vi "Database Recordset Open.vi"(6 "LockType":i32(ring)=-1 items=["adLockUnspecified"=-1, "adLockReadOnly"=1, "adLockPessimistic"=2, "adLockOptimistic"=3, "adLockBatchOptimistic"=4], 7 "CursorType":i32(ring)=-1 items=["adOpenUnspecified"=-1, "adOpenForwardOnly"=0, "adOpenKeyset"=1, "adOpenDynamic"=2, "adOpenStatic"=3], 8 "error in (no error)":errorcluster caption="错误输入（无错误）", 9 "Options":i32, 10 "Command Text":string, 11 "Database Recordset 输入":refnum<class "Database Recordset.lvclass"> caption="DNL_LabVIEW Object in") -> (0 "error out":errorcluster caption="错误输出", 3 "Database Recordset 输出":refnum<class "Database Recordset.lvclass"> caption="DNL_LabVIEW Object out")   [LabVIEW 2011, in "Database Recordset.lvclass"]
uses:
  Database Recordset.lvclass
  Database Recordset.lvclass/Database Recordset.ctl
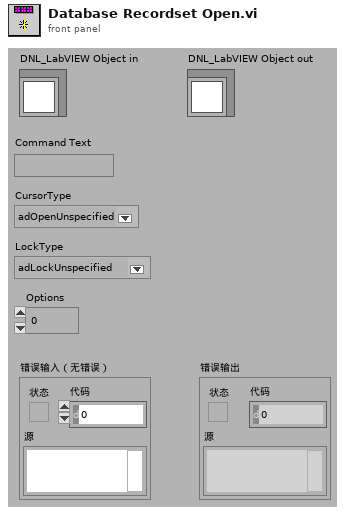
[diagram p1: front panel]
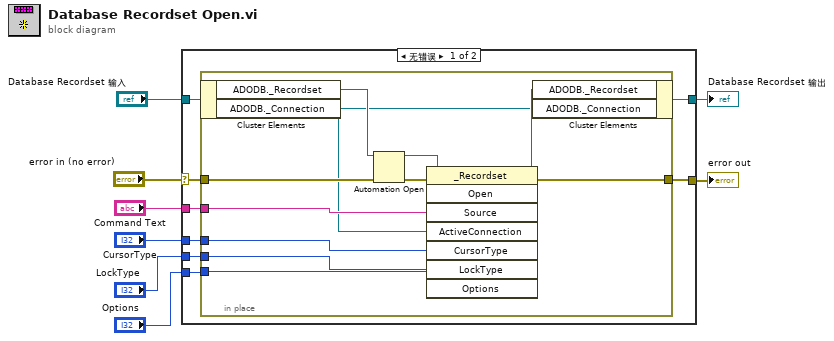
[diagram p0: block diagram]
diagram:
  n1 = case shown="无错误" "error in (no error)" {
    selector: "error in (no error)" -> [w14 w29]
    tunnel: [w9 w29] -> w7
    tunnel: [w15 w28] -> w5
    tunnel: "Database Recordset 输入" -> [w16 w28]
    tunnel: "Command Text" -> [w13 _]
    tunnel: "CursorType" -> [w12 _]
    tunnel: "Options" -> [w11 _]
    tunnel: "LockType" -> [w10 _]
    frame No Error {
      n2 = in-place {
        in-place-border: w14 -> [w24]
        in-place-border: w13 -> [w22]
        in-place-border: w12 -> [w21]
        in-place-border: w11 -> [w20]
        in-place-border: w10 -> [w19]
        in-place-border: [w18] -> w9
        n3 = in-place-cluster #1(w16) -> ("ADODB._Recordset"=w26:refnum<k7>, "ADODB._Connection"=w17:refnum<k7>)
        n4 = Automation Open(error in (no error)=w24, Automation Refnum=w26) -> (Automation Refnum=w27:refnum<k7>, error out=w23:errorcluster)  [unwired: 2 in]
        n5 = invoke class="_Recordset" method="Open"(reference=w27, error in=w23, "Source"=w22, "ActiveConnection"=w17, "CursorType"=w21, "LockType"=w19, "Options"=w20) -> (reference out=w25:refnum<k7>, error out=w18:errorcluster)  [unwired: 1 in, 6 out]
        n6 = in-place-cluster #1("ADODB._Recordset"=w25, "ADODB._Connection"=w17) -> (w15:refnum<class "Database Recordset.lvclass">)
      }
    }
    frame Error {
    }
  }
  "error out" <- w7
  "Database Recordset 输出" <- w5
